vi "Generate Local Event.vi"(8 "error in (no error)":errorcluster, 10 "Data":variant, 11 "Event Type":T1=enum."Button 0 Click") -> (0 "error out":errorcluster)   [LabVIEW 2019, in "GaitDAQ UI.lvlib"]
uses:
  GaitDAQ UI.lvlib
  Event/Event Type.ctl
  Event/GaitDAQ UI Event.lvlib
panel:
  # "Input"
  # "Output"
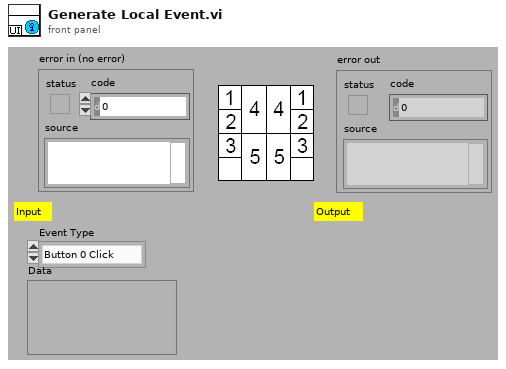
[diagram p1: front panel]
types:
  T1 = typedef "GaitDAQ UI Event.lvlib/Event Type.ctl" = enum16{"Default", "Initialize Finish", "Button 0 Click", "Panel Close", "Exit"}
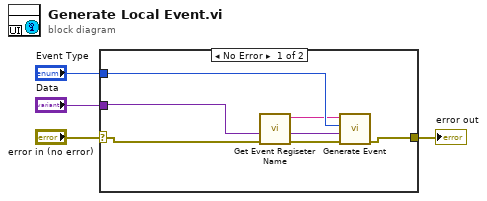
[diagram p0: block diagram]
diagram:
  n1 = case shown="No Error" "error in (no error)" {
    selector: "error in (no error)" -> [w5 w11]
    tunnel: [w8 w11] -> w3
    tunnel: "Data" -> [w10 _]
    tunnel: "Event Type" -> [w9 _]
    frame No Error {
      n2 = call "Get Event Regiseter Name.vi"("error in (no error)"=w5) -> ("error out"=w6:errorcluster, "Event Register Name"=w7:string)  [unwired: 9 in]
      n3 = call "Generate Event.vi"("error in (no error)"=w6, "Data"=w10, "Event Type"=w9, "Sender"=w7) -> ("error out"=w8:errorcluster)  [unwired: 7 in]
    }
    frame Error {
    }
  }
  "error out" <- w3
